vi "+-1V Conv.vi"(1 "Register Value":u16) -> (0 "Voltage V":dbl)   [LabVIEW 2024]
doc: "Convert analogue register value to +-1V value."
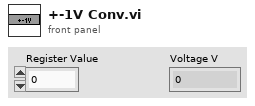
[diagram p1: front panel]
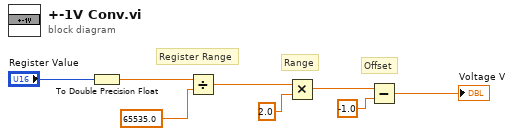
[diagram p0: block diagram]
diagram:
  # "Register Range"
  # "Offset"
  # "Range"
  n1 = To Double Precision Float(number="Register Value") -> (double precision float=w1:dbl)
  n2 = Divide(x=w1, y=65535.0) -> (x/y=w4:dbl)
  n3 = Multiply(x=w4, y=2.0) -> (x*y=w6:dbl)
  n4 = Subtract(x=w6, y=-1.0) -> (x-y=→"Voltage V":dbl)
